vi "fpga.sandbox.ip.vi"(0 "ip.reset":bool, 5 "TDATA":u64, 7 "TKEEP":u8, 9 "TUSER":bool, 11 "TVALID":bool, 12 "TLAST":bool) -> (4 "DEBUG.TDATA":u64, 6 "DEBUG.TKEEP":u8, 8 "DEBUG.TVALID":bool, 10 "DEBUG.TLAST":bool)   [LabVIEW 2025]
uses:
  <vilib>/Platform/TimedLoop/XDataNode/timing_clust.ctl
  <vilib>/Platform/TimedLoop/XDataNode/nitl_modes.ctl
  <vilib>/Platform/TimedLoop/XDataNode/wakeup.ctl
  submodules/Market.Data.Bats.Parser/fpga/poc.ip.debug.states.ctl
  <vilib>/rvi/Emulation/niFpgaSctlEmulationGetInTimedLoop.vi
  <vilib>/rvi/Emulation/niFpgaEmulationReportErrorSimple.vi
  <vilib>/rvi/Emulation/niFpgaGetClockAttributes.vi
  <vilib>/rvi/Emulation/niFpgaCriticalErrorInLSC.vi
  <vilib>/rvi/Emulation/niFpgaEmulationIsFPGAContextNoSignature.vi
  <vilib>/rvi/errors/niFpgaSetErrorForExecOnDevCompSimple.vi
  <vilib>/rvi/eio/common/nirviEmuReportErrorAndStop.vi
  <vilib>/rvi/DataTransferAndStorage/Container/Common/niFpgaContainerGetUniqueNameForEmu.vi
  <vilib>/rvi/FIFO/Fifo_Resource/nirvififoEmulationSetSize.vi
  <vilib>/rvi/FIFO/Fifo_Resource/nirviFifoEmulationQueueMgr.vi
  <instcachedir>/0/nirviFifoEmulationQueueMgr_E5CAEC123FF24DC58D834DCA3CDAA9B5.lvgen/nirviFifoEmulationQueueMgr_E5CAEC123FF24DC58D834DCA3CDAA9B5_002.vi
  <vilib>/Utility/error.llb/Clear Errors.vi
  <vilib>/rvi/FIFO/Fifo_Resource/nirvififoEmulationCreateLock.vi
  <vilib>/rvi/Emulation/niFpgaProcessEmulError.vi
  <vilib>/rvi/FIFO/Fifo_Resource/nirvififoEmulationObtainLock.vi
  <vilib>/rvi/FIFO/Fifo_Resource/nirvififoEmulationReleaseLock.vi
  <vilib>/rvi/occurrence/nirviWaitOnOccurrenceBase.vi
  <vilib>/rvi/errors/nirviReportUnexpectedCaseInternalError.vi
  <vilib>/rvi/errors/nirviReportUnexpectedCaseInternalError (U32).vi
  <vilib>/Platform/TimedLoop/XDataNode/XDataNode.xnode
  <vilib>/rvi/DataTransferAndStorage/Container/XNode/niFpgaContainer.xnode
  <vilib>/rvi/FIFO/Fifo_Resource/nirvififoEmulationRead.vi
  <vilib>/Platform/TimedLoop/XDataNode/XDNodeRunTimeDep.lvlib
  axi_2_eth_raw.ctl
  <vilib>/rvi/interface/RandomDataEmulation/nirviRandomDataFpgaMultiElementTemplate.vi
  <vilib>/rvi/Memory/Memory_Emulation/niFpgaMemoryEmulationRefIn.vi
  <vilib>/rvi/FIFO/Fifo_Resource/niFpgaFifoEmulationRefIn.vi
  <vilib>/rvi/LocalResourceManager/LocalResourceManager.xnode
  <vilib>/rvi/DataTransferAndStorage/Container/Common/niFpgaContainerSetEmuInfo.vi
  submodules/Market.Data.Bats.Parser/fpga/poc.ip.axi.write.states.ctl
panel:
  out "TREADY":bool
  in  "DEBUG.TREADY":bool
  out "Sum.Out":u8
  in  "B.in":u8
  in  "A.in":u8
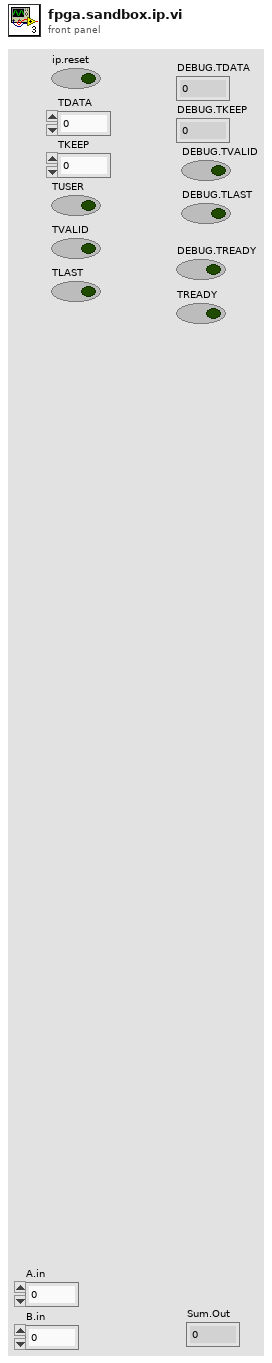
[diagram p1: front panel]
types:
  T1 = typedef "XDNodeRunTimeDep.lvlib/timing_clust.ctl" = cluster{"Expected End [f-1]":u64, "Actual End [f-1]":u64, "Finished Late? [f-1]":bool, "Expected End [i-1]":u64, "Actual End [i-1]":u64, "Finished Late? [i-1]":bool, "Expected Start [i]":u64, "Actual Start [i]":u64, "Expected Start [f]":u64, "Actual Start [f]":u64, "Source Name":string, "Structure Name":string, "Period":i64, "Deadline":i64, "Offset":i64, "Start":i64, "Priority":i32, "Timeout":i32, "Mode":T2, "Wakeup Reason":T3, "Error":errorcluster, "Source Type":string, "Secondary Source Type":string, "Global End Time":u64, "Global Start Time":u64, "Frame Duration":u64, "Iteration Duration":u64, "Assigned CPU":i32, "I/O Scan Engine Mode":u32}
  T2 = typedef "XDNodeRunTimeDep.lvlib/nitl_modes.ctl" = enum32{"No Change", "Process missed periods, maintain original phase", "Discard missed periods, maintain original phase", "Process missed periods, ignore original phase", "Discard missed periods, ignore original phase"}
  T3 = typedef "XDNodeRunTimeDep.lvlib/wakeup.ctl" = enum32{"Normal", "Aborted", "Asynchronous wakeup", "Timing source error", "Timed loop error", "Timeout"}
  T4 = typedef "poc.ip.axi.write.states.ctl" = enum16{"Wait", "Collect"}
  T5 = typedef "poc.ip.debug.states.ctl" = enum16{"Wait", "Write.Data"}
  T6 = cluster{"data valid":bool, "end.of.frame":bool, "start.of.frame":bool, "data":u64, "byte enables":u8}
  T7 = typedef "axi_2_eth_raw.ctl" = cluster{"data valid":bool, "end.of.frame":bool, "start.of.frame":bool, "data":u64, "byte enables":u8}
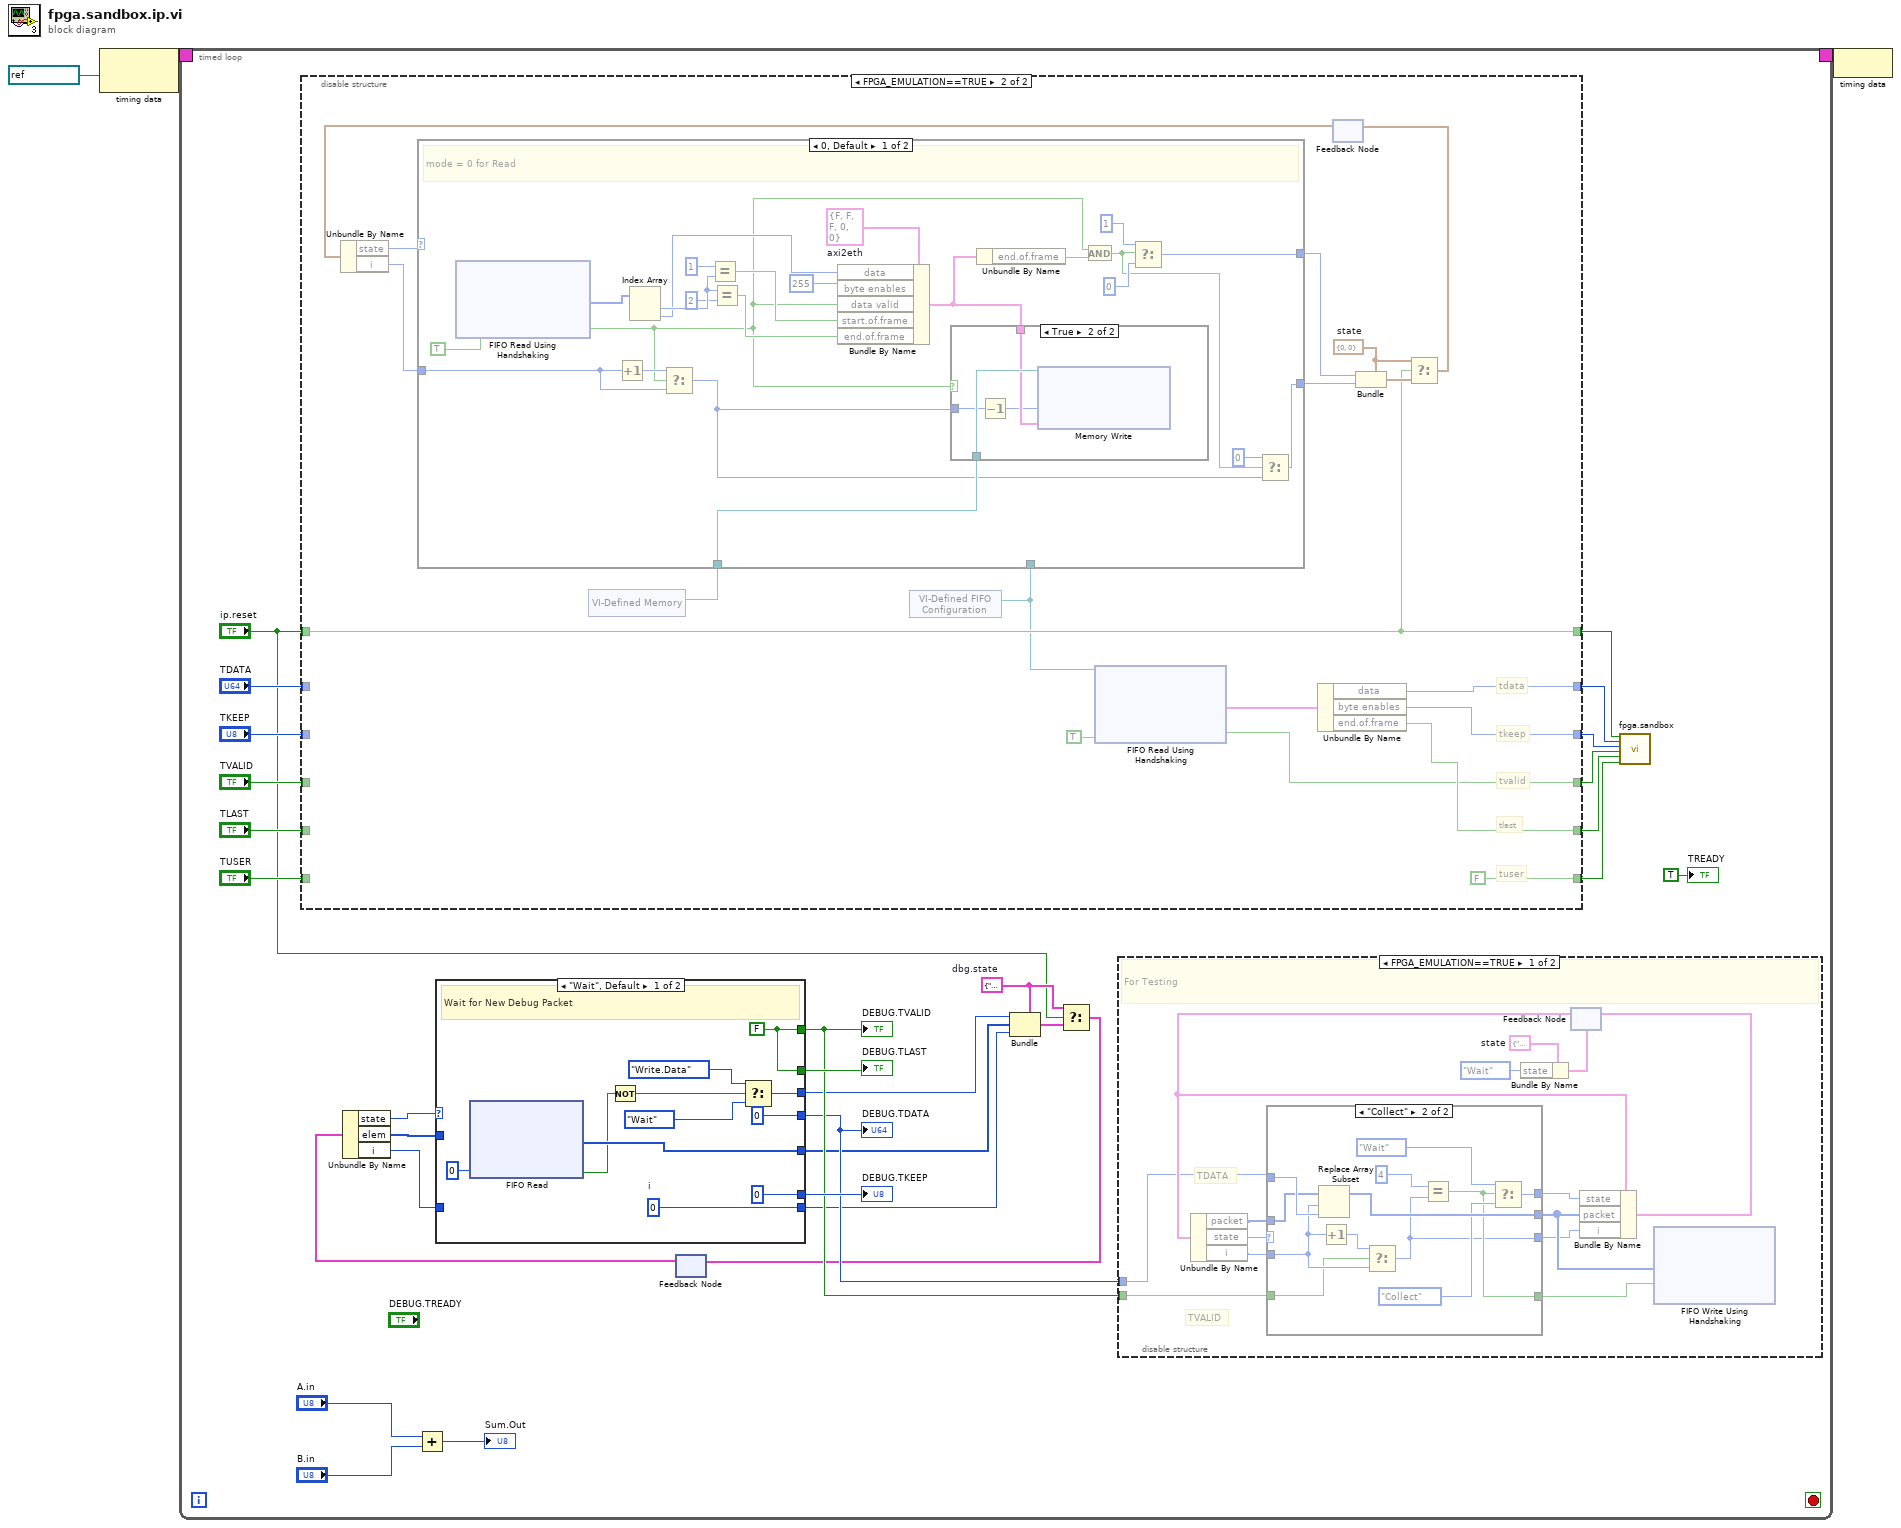
[diagram p0: block diagram]
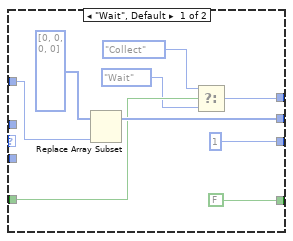
[diagram p2: hidden frame]
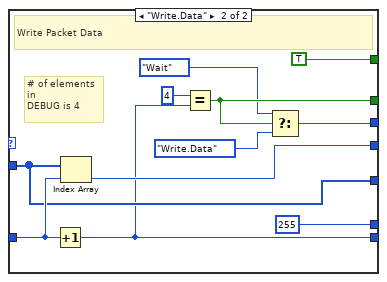
[diagram p4: hidden frame]
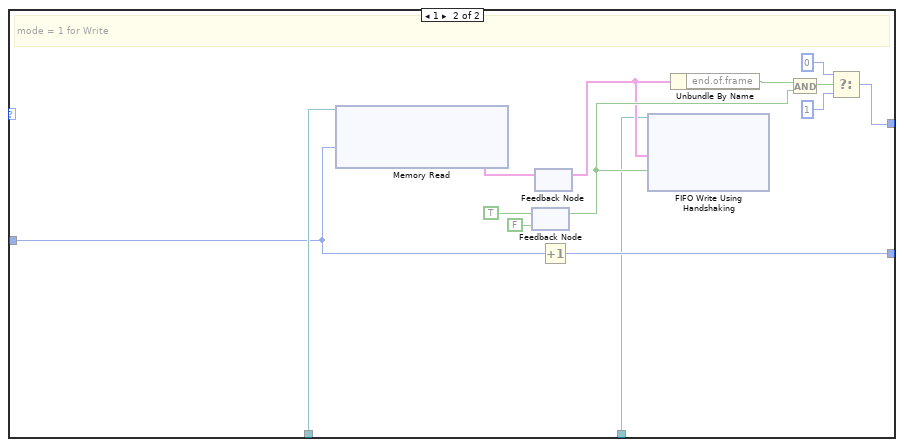
[diagram p7: hidden frame]
diagram:
  n1 = node-c288(refnum<k21> "100MHz" ("Source Name")) -> (w3:T1)
  n2 = timed-loop {
    timing: w3 -> [_]
    timing-out: [_] -> w2
    stop <- _ stop-if-true
    w18 = cluster{"state":T5, "elem":u64[], "i":i16} {"state"=enum."Wait", "elem"=[0, 0, 0, 0], "i"=0}  # dbg.state
    n3 = disable-structure shown="FPGA_EMULATION==TRUE" {
      disable-tunnel: [w96 w98] -> w12
      disable-tunnel: "TDATA" -> [w96 _]
      disable-tunnel: [w95 w97] -> w11
      disable-tunnel: "TKEEP" -> [w95 _]
      disable-tunnel: [w94 w99] -> w10
      disable-tunnel: "TVALID" -> [w94 _]
      disable-tunnel: [w93 w100] -> w9
      disable-tunnel: "TLAST" -> [w93 _]
      disable-tunnel: [w92 FALSE ("TUSER")] -> w8
      disable-tunnel: "TUSER" -> [w92 _]
      disable-tunnel: "ip.reset" -> [w91 w105]
      disable-tunnel: [w91 w105] -> w13
      frame condition #0 (active) {
      }
      frame condition #1 {
        w110 = cluster{"state":u8, "i":u16} {"state"=0, "i"=0}  # state
        # "tkeep"
        # "tdata"
        # "tuser"
        # "tlast"
        # "tvalid"
        n4 = xnode "VI-Defined Memory"() -> ("Memory Out"=w106:refnum<k21>)
        n5 = xnode "VI-Defined FIFO Configuration"() -> ("FIFO Out"=w102:refnum<k21>)
        n6 = xnode "FIFO Read Using Handshaking"("Ready for Output"=TRUE, "FIFO In"=w102) -> ("Element"=w103:T6, "Output Valid"=w99:bool)  [unwired: 1 out]
        n7 = Unbundle By Name(w103) -> ("data"=w98:u64, "byte enables"=w97:u8, "end.of.frame"=w100:bool)
        n8 = feedback #1() -> (w112:cluster{"state":u8, "i":u16})  [unwired: 1 in]
        n9 = Unbundle By Name(w112) -> ("state"=w113:u8, "i"=w114:u16)
        n10 = case shown="0, Default" w113 {
          tunnel: w114 -> [w126 w143]
          tunnel: w106 -> [w125 w155]
          tunnel: [w118 w149] -> w108
          tunnel: [w120 w152] -> w107
          tunnel: w102 -> [_ w142]
          frame 0, Default {
            w137 = T7 {"data valid"=FALSE, "end.of.frame"=FALSE, "start.of.frame"=FALSE, "data"=0, "byte enables"=0}  # axi2eth
            # "mode = 0 for Read"
            n11 = xnode "FIFO Read Using Handshaking"("Ready for Output"=TRUE) -> ("Element"=w136:u64[], "Output Valid"=w119:bool)  [unwired: 1 in, 1 out]
            n12 = Increment(x=w126) -> (x+1=w127:u16)
            n13 = Index Array(array=w136) -> (element #1=w135:u64, element #2=w129:u64)  [unwired: 2 in]
            n14 = Select(t=w127, s=w119, f=w126) -> (s? t:f=w117:u16)
            n15 = Equal?(x=u64 1, y=w135) -> (x = y?=w131:bool)
            n16 = Equal?(x=w135, y=u64 2) -> (x = y?=w132:bool)
            n17 = Bundle By Name(cluster=w137, "data"=w129, "byte enables"=u8 255 ("number"), "data valid"=w119, "start.of.frame"=w131, "end.of.frame"=w132) -> (w124:T7)
            n18 = case shown="True" w119 {
              tunnel: w125 -> [_ w141]
              tunnel: w124 -> [_ w140]
              tunnel: w117 -> [_ w139]
              frame False {
              }
              frame True {
                n19 = Decrement(x=w139) -> (x-1=w138:u16)
                n20 = xnode "Memory Write"("Address"=w138, "Data"=w140, "Memory In"=w141) -> ()  [unwired: 1 out]
              }
            }
            n21 = Unbundle By Name(w124) -> ("end.of.frame"=w123:bool)
            n22 = And(x=w119, y=w123) -> (x .and. y?=w116:bool)
            n23 = Select(t=u8 1, s=w116, f=u8 0 ("t")) -> (s? t:f=w120:u8)
            n24 = Select(t=u16 0, s=w116, f=w117) -> (s? t:f=w118:u16)
          }
          frame 1 {
            # "mode = 1 for Write"
            n25 = xnode "Memory Read"("Address"=w143, "Memory In"=w155) -> ("Data"=w154:T6)  [unwired: 1 out]
            n26 = feedback-in #2(TRUE ("Input Valid")) -> ()
            n27 = feedback #2(FALSE ("Input Valid")) -> (w145:bool)
            n28 = feedback-in #3(w154) -> ()
            n29 = feedback #3() -> (w144:T6)  [unwired: 1 in]
            n30 = Increment(x=w143) -> (x+1=w149:u16)
            n31 = xnode "FIFO Write Using Handshaking"("Element"=w144, "Input Valid"=w145, "FIFO In"=w142) -> ()  [unwired: 2 out]
            n32 = Unbundle By Name(w144) -> ("end.of.frame"=w153:bool)
            n33 = And(x=w153, y=w145) -> (x .and. y?=w146:bool)
            n34 = Select(t=u8 0 ("f"), s=w146, f=u8 1) -> (s? t:f=w152:u8)
          }
        }
        n35 = Bundle(cluster=w110, "state"=w107, "i"=w108) -> (w109:cluster{"state":u8, "i":u16})
        n36 = Select(t=w110, s=w105, f=w109) -> (s? t:f=w111:cluster{"state":u8, "i":u16})
        n37 = feedback-in #1(w111) -> ()
      }
    }
    n38 = Add(x="A.in", y="B.in") -> (x+y=→"Sum.Out":u8)
    n39 = feedback #4() -> (w19:cluster{"state":T5, "elem":u64[], "i":i16})  [unwired: 1 in]
    n40 = Unbundle By Name(w19) -> ("state"=w17:T5, "elem"=w16:u64[], "i"=w15:i16)
    n41 = case shown="\"Wait\", Default" w17 {
      tunnel: [w77 w85] -> w22
      tunnel: w15 -> [_ w90]
      tunnel: [w79 w82] -> w24
      tunnel: [w78 w89] -> w23
      tunnel: w16 -> [_ w89]
      tunnel: [u64 0 ("Data") w88] -> w25
      tunnel: [u8 0 ("DEBUG.TKEEP") u8 255 ("DEBUG.TKEEP")] -> w28
      tunnel: [w76 w83] -> w27
      tunnel: [w76 TRUE] -> w26
      frame "Wait", Default {
        w76 = FALSE
        w77 = i16 0  # i
        # "Wait for New Debug Packet"
        n42 = xnode ("FIFO Read")("Timeout"=0) -> ("Element"=w78:u64[], "Timed Out?"=w69:bool)  [unwired: 1 in, 1 out]
        n43 = Not(x=w69) -> (.not. x?=w71:bool)
        n44 = Select(t=poc.ip.debug.states."Write.Data", s=w71, f=poc.ip.debug.states."Wait") -> (s? t:f=w79:T5)
      }
      frame "Write.Data" {
        # "# of elements \nin \nDEBUG is 4"
        # "Write Packet Data"
        n45 = Increment(x=w90) -> (x+1=w85:i16)
        n46 = Index Array(array=w89, index=w90) -> (element=w88:u64)
        n47 = Equal?(x=i16 4, y=w85) -> (x = y?=w83:bool)
        n48 = Select(t=poc.ip.debug.states."Wait", s=w83, f=poc.ip.debug.states."Write.Data") -> (s? t:f=w82:T5)
      }
    }
    "DEBUG.TDATA" <- w25
    "DEBUG.TKEEP" <- w28
    "DEBUG.TVALID" <- w26
    "DEBUG.TLAST" <- w27
    n49 = Bundle(cluster=w18, "state"=w24, "elem"=w23, "i"=w22) -> (w21:cluster{"state":T5, "elem":u64[], "i":i16})
    n50 = Select(t=w18, s="ip.reset", f=w21) -> (s? t:f=w20:cluster{"state":T5, "elem":u64[], "i":i16})
    n51 = feedback-in #4(w20) -> ()
    n52 = disable-structure shown="FPGA_EMULATION==TRUE" {
      disable-tunnel: w26 -> [w35 _]
      disable-tunnel: w25 -> [w34 _]
      frame condition #0 {
        w36 = cluster{"state":T4, "packet":u64[], "i":u16} {"state"=enum."Wait", "packet"=[0, 0, 0, 0], "i"=0}  # state
        # "TVALID"
        # "TDATA"
        # "For Testing"
        n53 = Bundle By Name(cluster=w36, "state"=poc.ip.axi.write.states."Wait" ("Enum")) -> (w40:cluster{"state":T4, "packet":u64[], "i":u16})
        n54 = feedback #5(w40) -> (w41:cluster{"state":T4, "packet":u64[], "i":u16})
        n55 = Unbundle By Name(w41) -> ("packet"=w46:u64[], "state"=w37:T4, "i"=w45:u16)
        n56 = case shown="\"Collect\"" w37 {
          tunnel: [FALSE w62] -> w38
          tunnel: [w48 w61] -> w43
          tunnel: w35 -> [w50 w58]
          tunnel: w34 -> [w53 w68]
          tunnel: [u16 1 ("i") w57] -> w44
          tunnel: [w52 w66] -> w47
          tunnel: w45 -> [_ w59]
          tunnel: w46 -> [_ w67]
          frame "Wait", Default {
            n57 = Replace Array Subset(array=u64[] [0, 0, 0, 0] ("packet"), new element=w53) -> (w52:u64[])  [unwired: 1 in]
            n58 = Select(t=poc.ip.axi.write.states."Collect" ("state"), s=w50, f=poc.ip.axi.write.states."Wait" ("state")) -> (s? t:f=w48:T4)
          }
          frame "Collect" {
            n59 = Replace Array Subset(array=w67, new element=w68, index=w59) -> (w66:u64[])
            n60 = Increment(x=w59) -> (x+1=w60:u16)
            n61 = Select(t=w60, s=w58, f=w59) -> (s? t:f=w57:u16)
            n62 = Equal?(x=u16 4, y=w57) -> (x = y?=w62:bool)
            n63 = Select(t=poc.ip.axi.write.states."Wait" ("Enum"), s=w62, f=poc.ip.axi.write.states."Collect" ("Enum")) -> (s? t:f=w61:T4)
          }
        }
        n64 = Bundle By Name(cluster=w41, "state"=w43, "packet"=w47, "i"=w44) -> (w42:cluster{"state":T4, "packet":u64[], "i":u16})
        n65 = feedback-in #5(w42) -> ()
        n66 = xnode "FIFO Write Using Handshaking"("Element"=w47, "Input Valid"=w38) -> ()  [unwired: 1 in, 2 out]
      }
      frame condition #1 (active) {
      }
    }
    n67 = call "fpga.sandbox.vi"("ip.reset"=w13, "TDATA"=w12, "TKEEP"=w11, "TVALID"=w10, "TLAST"=w9, "TUSER"=w8) -> ()  [unwired: 14 in]
    "TREADY" <- TRUE ("TREADY")
  }
  n68 = node-c288(w2) -> ()
